vi "Update ChnlInterruptBit.vi"(8 "error in (no error)":errorcluster, 9 "current time":timestamp, 10 "InterruptBits":i32, 11 "BME_DG_Chnl in":refnum<class "BME_DG_Chnl.lvclass">) -> (0 "error out":errorcluster, 1 "ShotPeriode":dbl, 2 "ChnlBit":bool, 3 "BME_DG_Chnl out":refnum<class "BME_DG_Chnl.lvclass">)   [LabVIEW 2009, in "POLARIS BME DG.lvlib" / "BME_DG_Chnl.lvclass"]
uses:
  BME_DG_Chnl.lvclass
  BME_DG_Chnl.lvclass/BME_DG_Chnl.ctl
  POLARIS BME DG.lvlib
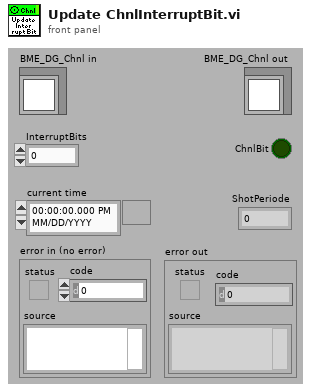
[diagram p1: front panel]
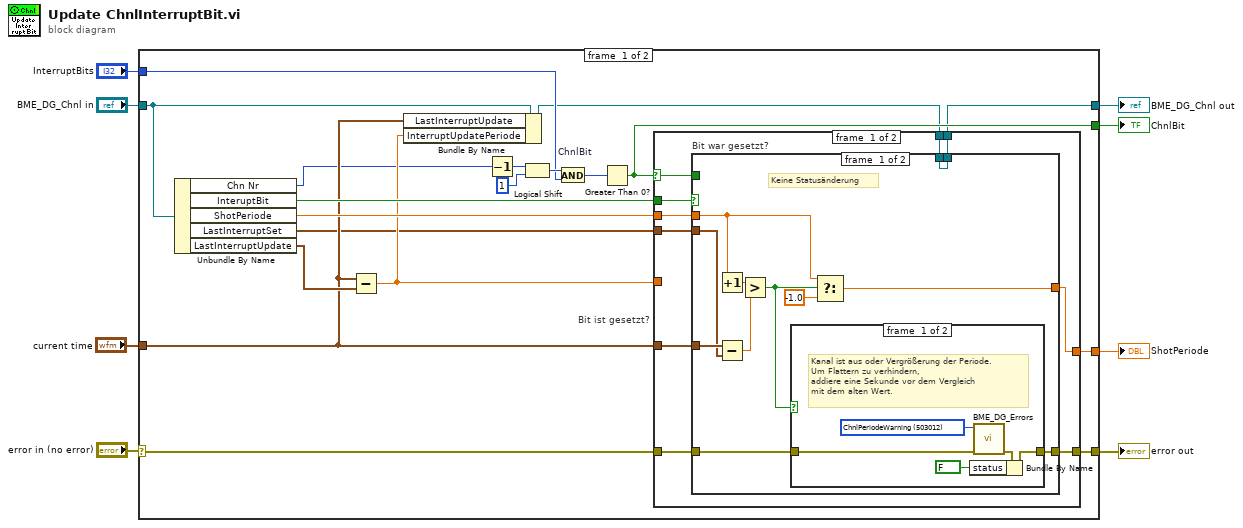
[diagram p0: block diagram]
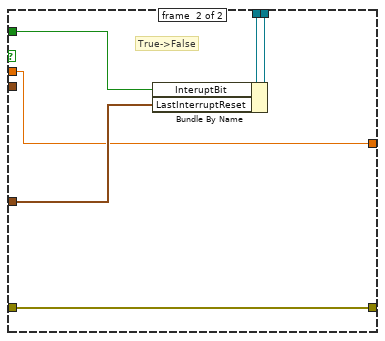
[diagram p3: hidden frame]
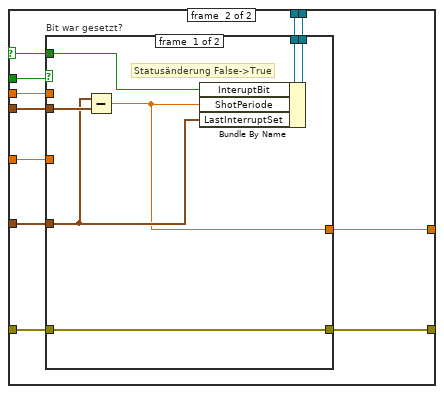
[diagram p4: hidden frame]
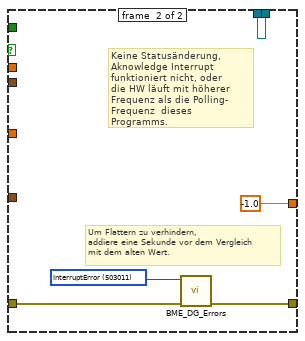
[diagram p5: hidden frame]
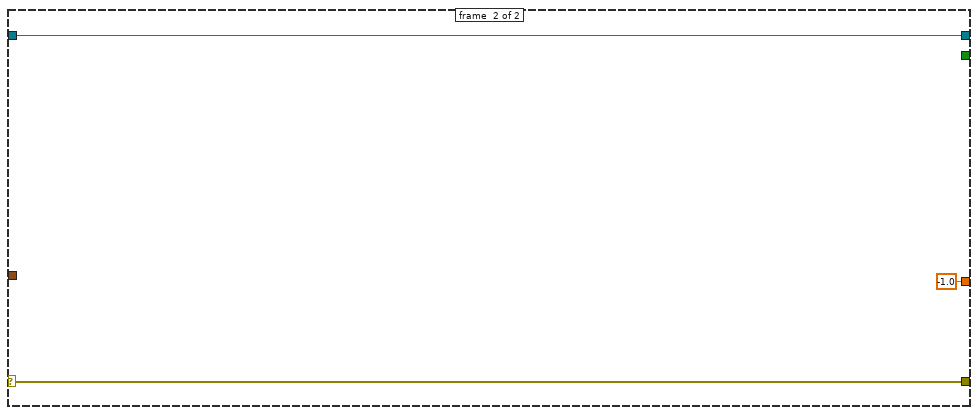
[diagram p6: hidden frame]
diagram:
  n1 = case shown="No Error" "error in (no error)" {
    selector: "error in (no error)" -> [w16 w84]
    tunnel: "BME_DG_Chnl in" -> [w27 w86]
    tunnel: "InterruptBits" -> [w23 _]
    tunnel: [w21 _] -> w6
    tunnel: [w20 w86] -> w5
    tunnel: "current time" -> [w12 _]
    tunnel: [w17 -1.0 ("f")] -> w3
    tunnel: [w15 w84] -> w1
    frame #0 {
      n2 = Unbundle By Name(w27) -> ("Chn Nr"=w9:i32, "InteruptBit"=w18:bool, "ShotPeriode"=w19:dbl, "LastInterruptSet"=w10:timestamp, "LastInterruptUpdate"=w13:timestamp)
      n3 = Subtract(x=w12, y=w13) -> (x-y=w11:dbl)
      n4 = Bundle By Name(cluster=w27, "LastInterruptUpdate"=w12, "InterruptUpdatePeriode"=w11) -> (w14:refnum<class "BME_DG_Chnl.lvclass">)
      n5 = Decrement(x=w9) -> (x-1=w25:i32)
      n6 = Logical Shift(y=w25, x=1) -> (x << y=w24:i32)
      n7 = And "ChnlBit"(x=w24, y=w23) -> (x .and. y?=w22:i32)
      n8 = Greater Than 0?(x=w22) -> (x > 0?=w21:bool)
      n9 = case "Bit ist gesetzt?" shown="False" w21 {
        selector: w21 -> [w35 w69]
        tunnel: w12 -> [w34 w68]
        tunnel: w14 -> [w37 w71]
        tunnel: [w36 w70] -> w20
        tunnel: w19 -> [w33 w66]
        tunnel: w18 -> [w31 w67]
        tunnel: [w32 w65] -> w17
        tunnel: w16 -> [w29 w64]
        tunnel: [w28 w63] -> w15
        tunnel: w11 -> [_ w62]
        tunnel: w10 -> [w30 w61]
        frame #0 {
          n10 = case "Bit war gesetzt?" shown="False" w31 {
            tunnel: w37 -> [w44 w60]
            tunnel: [w44 w57] -> w36
            tunnel: w35 -> [_ w59]
            tunnel: w34 -> [w47 w58]
            tunnel: w33 -> [w43 w56]
            tunnel: [w41 w56] -> w32
            tunnel: w30 -> [w46 _]
            tunnel: w29 -> [w40 w55]
            tunnel: [w39 w55] -> w28
            frame #0 {
              # "Keine Statusänderung"
              n11 = Increment(x=w43) -> (x+1=w45:dbl)
              n12 = Subtract(x=w47, y=w46) -> (x-y=w42:dbl)
              n13 = Greater?(x=w45, y=w42) -> (0:w38:bool)
              n14 = case shown="False" w38 {
                tunnel: w40 -> [w53 w54]
                tunnel: [w51 w54] -> w39
                frame #0 {
                  w49 = 503012 items=["Channel refers itself"=503001, "Deadloop"=503002, "Negative Delay"=503003, "Delay Card not found"=503004, "Channel not found"=503005, "Parse Error"=503006, "Not Supported"=503007, "Systen not found"=503008, "To much masters"=503009, "None master in Syterm"=503010, "InterruptError"=503011, "ChnlPeriodeWarning"=503012] ("error")
                  # "Kanal ist aus oder Vergrößerung der Periode.\nUm Flattern zu verhindern,\naddiere eine Sekunde vor dem Vergleich\nmit dem alten Wert."
                  n15 = call "BME_DG_Errors.vi"("error in (no error)"=w53, "error"=w49) -> ("error out"=w52:errorcluster)  [unwired: 9 in]
                  n16 = Bundle By Name(cluster=w52, "status"=FALSE) -> (w51:errorcluster)
                }
                frame #1 {
                }
              }
              n17 = Select(t=w43, s=w38, f=-1.0) -> (s? t:f=w41:dbl)
            }
            frame #1 {
              # "True->False"
              n18 = Bundle By Name(cluster=w60, "InteruptBit"=w59, "LastInterruptReset"=w58) -> (w57:refnum<class "BME_DG_Chnl.lvclass">)
            }
          }
        }
        frame #1 {
          n19 = case "Bit war gesetzt?" shown="True" w67 {
            tunnel: w71 -> [w78 w83]
            tunnel: [w77 w83] -> w70
            tunnel: w69 -> [w76 _]
            tunnel: w68 -> [w73 _]
            tunnel: w66 -> [_ _]
            tunnel: [w72 -1.0 ("f")] -> w65
            tunnel: w64 -> [w75 w81]
            tunnel: [w75 w80] -> w63
            tunnel: w62 -> [_ _]
            tunnel: w61 -> [w74 _]
            frame #0 {
              # "Statusänderung False->True"
              n20 = Subtract(x=w73, y=w74) -> (x-y=w72:dbl)
              n21 = Bundle By Name(cluster=w78, "InteruptBit"=w76, "ShotPeriode"=w72, "LastInterruptSet"=w73) -> (w77:refnum<class "BME_DG_Chnl.lvclass">)
            }
            frame #1 {
              w82 = 503011 items=["Channel refers itself"=503001, "Deadloop"=503002, "Negative Delay"=503003, "Delay Card not found"=503004, "Channel not found"=503005, "Parse Error"=503006, "Not Supported"=503007, "Systen not found"=503008, "To much masters"=503009, "None master in Syterm"=503010, "InterruptError"=503011] ("error")
              # "Um Flattern zu verhindern,\naddiere eine Sekunde vor dem Vergleich\nmit dem alten Wert."
              # "Keine Statusänderung,\nAknowledge Interrupt\nfunktioniert nicht, oder\ndie HW läuft mit höherer\nFrequenz als die Polling-\nFrequenz  dieses Programms."
              n22 = call "BME_DG_Errors.vi"("error in (no error)"=w81, "error"=w82) -> ("error out"=w80:errorcluster)  [unwired: 9 in]
            }
          }
        }
      }
    }
    frame #1 {
    }
  }
  "error out" <- w1
  "BME_DG_Chnl out" <- w5
  "ChnlBit" <- w6
  "ShotPeriode" <- w3
